vi "Transmit.vi"(8 "error in (no error)":errorcluster, 10 "Transfer Group in":refnum<class "Transfer Group.lvclass">, 11 "UDP Transceiver in":refnum<class "DSF UDP Transceiver.lvclass">) -> (0 "error out":errorcluster, 2 "Transfer Group out":refnum<class "Transfer Group.lvclass">, 3 "UDP Transceiver out":refnum<class "DSF UDP Transceiver.lvclass">)   [LabVIEW 2017, in "DSF Core.lvlib" / "DSF UDP Transceiver.lvclass"]
uses:
  DSF UDP Transceiver.lvclass
  Classes/Transfer Group/Transfer Group.lvclass
  DSF UDP Transceiver.lvclass/DSF UDP Transceiver.ctl
  Write Datagram to Port.vi
  <vilib>/Utility/error.llb/Clear Errors.vi
  Classes/Transfer Group/Get Active Buffer.vi
  Classes/Buffer/Get Buffer Size.vi
  Classes/Buffer/Read Buffer.vi
  Classes/Buffer/Read Buffer 1D U8.vi
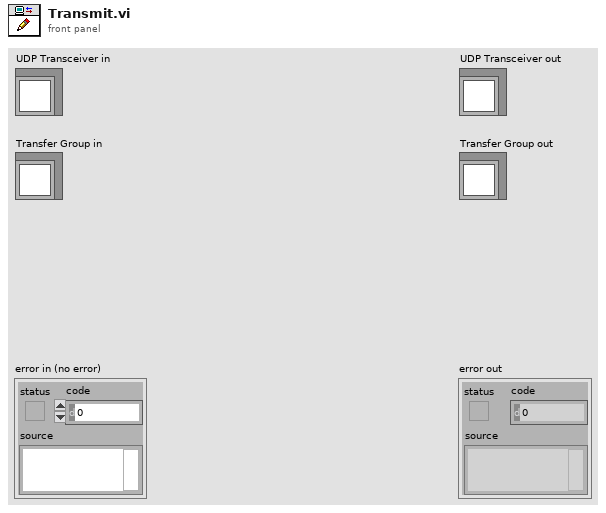
[diagram p1: front panel]
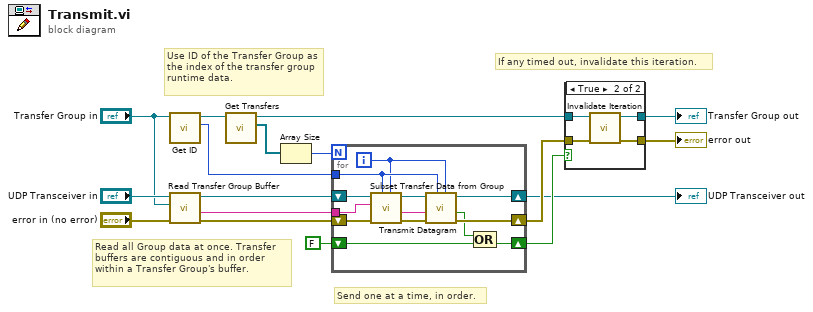
[diagram p0: block diagram]
diagram:
  # "If any timed out, invalidate this iteration."
  # "Send one at a time, in order."
  # "Read all Group data at once. Transfer buffers are contiguous and in order within a Transfer Group's buffer."
  # "Use ID of the Transfer Group as the index of the transfer group runtime data."
  n1 = call "Get ID.vi"("Transfer Group in"="Transfer Group in") -> ("id"=w17:i32, "Transfer Group out"=w8:refnum<class "Transfer Group.lvclass">)  [unwired: 9 in]
  n2 = call "Read Transfer Group Buffer.vi"("error in (no error)"="error in (no error)", "Transfer Group"="Transfer Group in", "UDP Transceiver in"="UDP Transceiver in") -> ("error out"=w12:errorcluster, "data"=w10:string, "UDP Transceiver out"=w11:refnum<class "DSF UDP Transceiver.lvclass">)  [unwired: 6 in]
  n3 = call "Get Transfers.vi"("Transfer Group in"=w8) -> ("Transfers"=w16:refnum<class "Transfer.lvclass">[], "Transfer Group out"=w6:refnum<class "Transfer Group.lvclass">)  [unwired: 9 in]
  n4 = Array Size(array=w16) -> (size(s)=w15:i32)
  n5 = for {
    N: w15 -> [_]
    shift-right: [w30] -> w4
    shift-left: w12 -> [w27]
    shift-right: [w18] -> w1
    shift-left: w11 -> [w29]
    tunnel: w17 -> [w24]
    tunnel: w10 -> [w22]
    shift-right: [w19] -> w2
    shift-left: FALSE -> [w21]
    i -> [w23]
    n6 = call "Subset Transfer Data from Group.vi"("transfer id"=w23, "transfer group id"=w24, "error in (no error)"=w27, "group data in"=w22, "UDP Transceiver in"=w29) -> ("error out"=w26:errorcluster, "transfer data"=w25:string, "UDP Transceiver out"=w28:refnum<class "DSF UDP Transceiver.lvclass">)  [unwired: 3 in, 1 out]
    n7 = call "Transmit Datagram.vi"("transfer id"=w23, "transfer group id"=w24, "error in (no error)"=w26, "transfer data"=w25, "UDP Transceiver in"=w28) -> ("error out"=w30:errorcluster, "timed out?"=w20:bool, "UDP Transceiver out"=w18:refnum<class "DSF UDP Transceiver.lvclass">)  [unwired: 4 in]
    n8 = Compound Arithmetic op=OR(w20, w21) -> (w19:bool)
  }
  "UDP Transceiver out" <- w1
  n9 = case shown="True" w2 {
    tunnel: w6 -> [w31 w36]
    tunnel: [w31 w35] -> w5
    tunnel: w4 -> [w32 w34]
    tunnel: [w32 w33] -> w3
    frame False {
    }
    frame True {
      n10 = call "Invalidate Iteration.vi"("error in (no error)"=w34, "Transfer Group in"=w36) -> ("error out"=w33:errorcluster, "Transfer Group out"=w35:refnum<class "Transfer Group.lvclass">)  [unwired: 8 in]
    }
  }
  "error out" <- w3
  "Transfer Group out" <- w5
